vi "CNR compute leverages.vi"(8 "error in (no error)":errorcluster, 10 "weight":dbl[](array[numeric]), 11 "J":T1) -> (0 "error out":errorcluster, 3 "leverages":dbl[](array[numeric]))   [LabVIEW 2018, in "NI_Gmath.lvlib"]
uses:
  NI_Gmath.lvlib
  RealMatrix.ctl
  Real A x B.vi
  Real PseudoInverse Matrix.vi
  <vilib>/Analysis/NI_AALBase.lvlib
  <vilib>/Analysis/NI_AALPro.lvlib
  NI_Matrix.lvlib
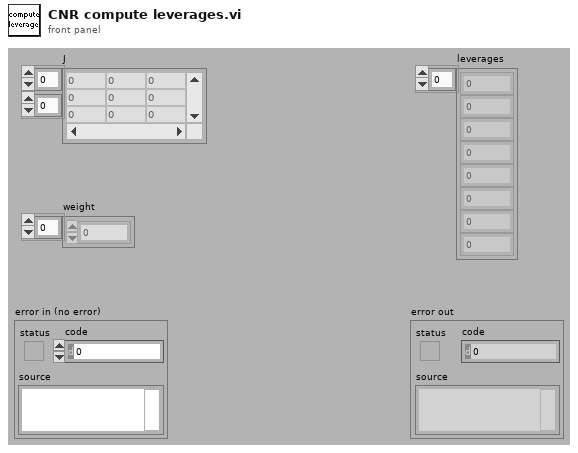
[diagram p1: front panel]
types:
  T1 = typedef "NI_Matrix.lvlib/RealMatrix.ctl" = dbl[][]
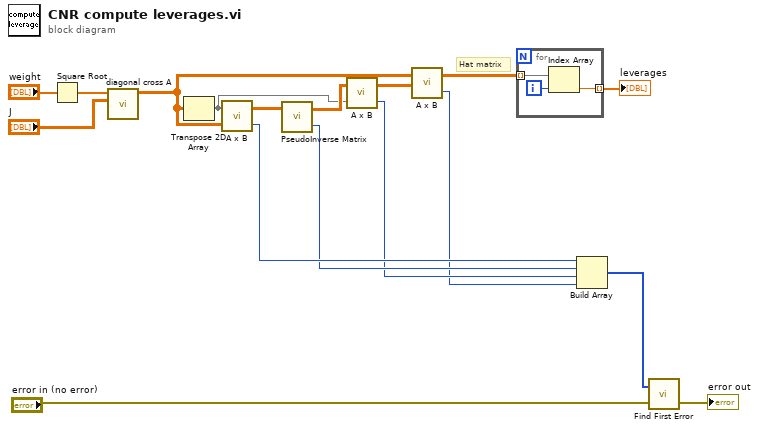
[diagram p0: block diagram]
diagram:
  # "Hat matrix"
  n1 = Square Root(x="weight") -> (sqrt(x)=w15:dbl[])
  n2 = call "diagonal cross A.vi"("A"="J", "diagonal"=w15) -> ("diagonalxA"=w13:T1)  [unwired: 9 in]
  n3 = Transpose 2D Array(2D array=w13) -> (transposed array=w1:T1)
  n4 = call-poly "A x B.vi"("B"=w13, "A"=w1) -> ("error"=w7:i32, "A x B"=w14:T1)
  n5 = call-poly "PseudoInverse Matrix.vi"("Input Matrix"=w14) -> ("error"=w6:i32, "PseudoInverse Matrix"=w2:T1)  [unwired: 1 in]
  n6 = call-poly "A x B.vi"("B"=w1, "A"=w2) -> ("error"=w5:i32, "A x B"=w12:T1)
  n7 = call-poly "A x B.vi"("B"=w12, "A"=w13) -> ("error"=w4:i32, "A x B"=w11:T1)
  n8 = for {
    tunnel: w11 -> [w20] mode=indexing
    tunnel: [w18] -> w10 mode=indexing
    i -> [w19]
    n9 = Index Array(array=w20, index=w19) -> (element=w18:dbl)
  }
  "leverages" <- w10
  n10 = Build Array(w7, w6, w5, w4) -> (w3:i32[])
  n11 = call "Find First Error.vi"("error in (no error)"="error in (no error)", "error codes"=w3) -> ("error out"=→"error out":errorcluster)  [unwired: 2 in, 1 out]
